vi "event.vi"() -> ()   [LabVIEW 2026]
panel:
  out "current time":timestamp
  out "Numeric":i32
  in  "stop":bool
  in  "OK Button":bool
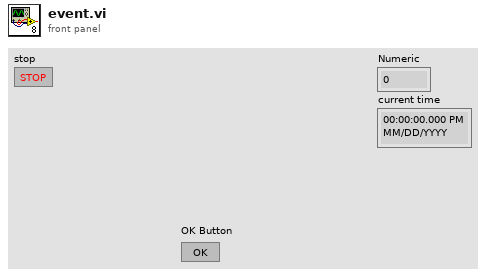
[diagram p1: front panel]
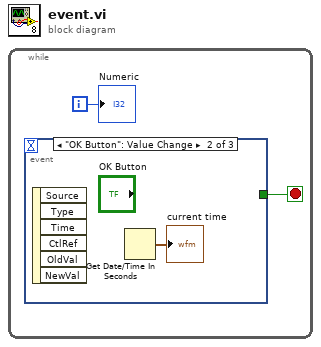
[diagram p0: block diagram]
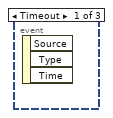
[diagram p2: hidden frame]
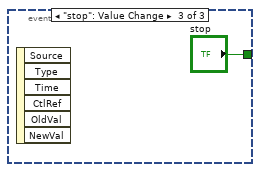
[diagram p3: hidden frame]
diagram:
  n1 = while {
    i -> [w2]
    stop <- w1 stop-if-true
    n2 = event shown="[1] \"OK Button\": Value Change" {
      selector: _ -> [_ _ _]
      dyn-events: _ -> [_ _ _]
      timeout: _ -> [_ _ _]
      tunnel: [_ _ "stop"] -> w1
      event Timeout {
        n3 = event-data() -> ()  [unwired: 1 in, 3 out]
      }
      event "OK Button": Value Change {
        n4 = event-data() -> ()  [unwired: 1 in, 6 out]
        n5 = Get Date/Time In Seconds() -> (seconds since 1Jan1904=→"current time":timestamp)
      }
      event "stop": Value Change {
        n6 = event-data() -> ()  [unwired: 1 in, 6 out]
      }
    }
    "Numeric" <- w2
  }
